vi "Array Indicies from Mouse.vi"(8 "error in (no error)":errorcluster, 11 "Array in":refnum<vi>) -> (0 "error out":errorcluster, 3 "Indicies":T1)   [LabVIEW 2017]
uses:
  <vilib>/Utility/miscctls.llb/LVBoundsTypeDef.ctl
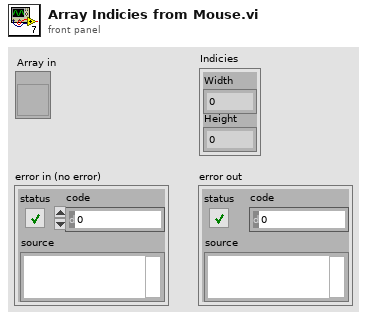
[diagram p1: front panel]
types:
  T1 = typedef "LVBoundsTypeDef.ctl" = cluster{"Width":u32, "Height":u32}
  T2 = typedef "LVPositionTypeDef.ctl" = cluster{"Left":i32, "Top":i32}
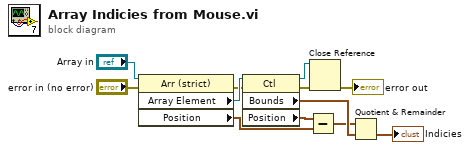
[diagram p0: block diagram]
diagram:
  n1 = property class="Arr (strict)"(reference="Array in", error in="error in (no error)") -> (error out=w8:errorcluster, "Array Element"=w9:refnum<vi>, "Position"=w2:T2)  [unwired: 1 out]
  n2 = property class="Ctl"(reference=w9, error in=w8) -> (reference out=w11:refnum<vi>, error out=w10:errorcluster, "Bounds"=w5:T1, "Position"=w3:T2)
  n3 = Subtract(x=w3, y=w2) -> (x-y=w4:T2)
  n4 = Close Reference(reference=w11, error in (no error)=w10) -> (error out=→"error out":errorcluster)
  n5 = Quotient & Remainder(x=w4, y=w5) -> (floor(x/y)=→"Indicies":T1)  [unwired: 1 out]
